vi "SetChanMode.vi"(8 "ChanMode":u8=1, 11 "错误输入":errorcluster) -> (3 "错误输出":errorcluster)   [LabVIEW 2016]
uses:
  PLC-Lab/lib/gusb.dll
panel:
  # "1：单端输入\n0：差分输入"
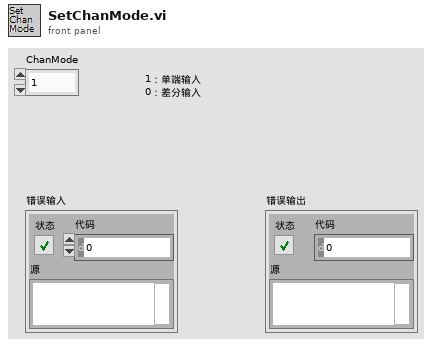
[diagram p1: front panel]
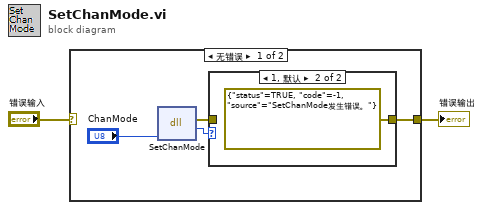
[diagram p0: block diagram]
diagram:
  n1 = case shown="无错误" "错误输入" {
    selector: "错误输入" -> [_ w9]
    tunnel: [w3 w9] -> w1
    frame No Error {
      n2 = dll-call lib="E:/Camproject/2018/2018.1Labview/PLC-Lab/lib/gusb.dll" fn="SetChanMode"("ChanMode"="ChanMode") -> (error out=w4:errorcluster, "Status"=w5:i32)  [unwired: 4 in, 1 out]
      n3 = case shown="1, 默认" w5 {
        tunnel: w4 -> [w7 _]
        tunnel: [w7 errorcluster {"status"=TRUE, "code"=-1, "source"="SetChanMode发生错误。"} ("错误常量")] -> w3
        frame 0 {
        }
        frame 1, Default {
        }
      }
    }
    frame Error {
    }
  }
  "错误输出" <- w1
